vi "Draw All Joints.vi"(8 "error out":errorcluster, 11 "Image":T1) -> (0 "error out 2":errorcluster, 3 "Image Out":T1)   [LabVIEW 2014]
uses:
  <vilib>/vision/Image Controls.llb/IMAQ Image.ctl
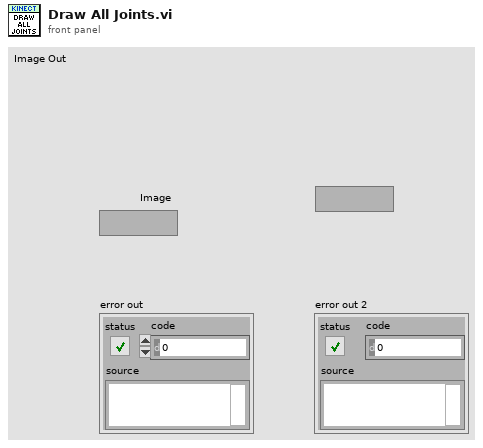
[diagram p1: front panel]
types:
  T1 = typedef "IMAQ Image.ctl" = refnum<image>
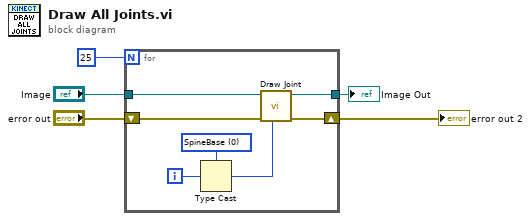
[diagram p0: block diagram]
diagram:
  n1 = for {
    N: 25 -> [_]
    shift-right: [w9] -> w2
    shift-left: "error out" -> [w8]
    tunnel: "Image" -> [w7]
    tunnel: [w6] -> w1
    i -> [w12]
    w11 = 0 items=["SpineBase", "SpineMid", "Neck", "Head", "ShoulderLeft", "ElbowLeft", "WristLeft", "HandLeft", "ShoulderRight", "ElbowRight", "WristRight", "HandRight", "HipLeft", "KneeLeft", "AnkleLeft", "FootLeft", "HipRight", "KneeRight", "AnkleRight", "FootRight", "SpineShoulder", "HandTipLeft", "ThumbLeft", "HandTipRight", "ThumbRight"] ("JointType")
    n2 = Type Cast(type=w11, x=w12) -> (*(type *) &x=w10:i32)
    n3 = call "Draw Joint.vi"("JointType"=w10, "error in"=w8, "Image"=w7) -> ("error out"=w9:errorcluster, "Image Out"=w6:T1)  [unwired: 7 in]
  }
  "error out 2" <- w2
  "Image Out" <- w1
